vi "发送测试脚本.vi"(7 "Script Name":string="TSB_Script", 8 "错误输入":errorcluster, 10 "Script":string, 11 "VISA资源名称":refnum<visa-resource-name>) -> (0 "错误输出":errorcluster, 3 "VISA资源名称输出":refnum<visa-resource-name>)   [LabVIEW 2021]
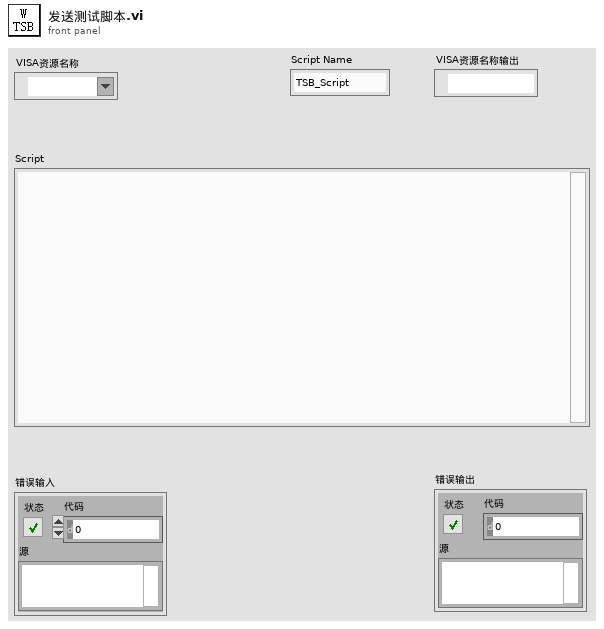
[diagram p1: front panel]
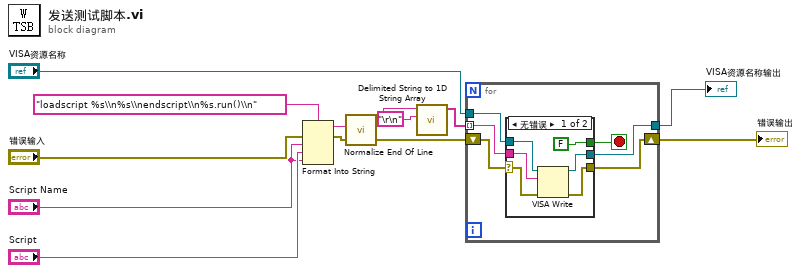
[diagram p0: block diagram]
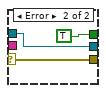
[diagram p2: hidden frame]
diagram:
  n1 = Format Into String(format string="loadscript %s\\n%s\\nendscript\\n%s.run()\\n", error in="错误输入", "Script Name", "Script", "Script Name") -> (resulting string=w4:string, error out=w1:errorcluster)  [unwired: 1 in]
  n2 = call <vilib>:"Normalize End Of Line.vi"("string in"=w4) -> ("string out"=w5:string)  [unwired: 7 in]
  n3 = call <vilib>:"Delimited String to 1D String Array.vi"("delimiter"="\r\n", "delimited string"=w5) -> ("string array"=w3:string[])  [unwired: 9 in]
  n4 = for {
    tunnel: "VISA资源名称" -> [w18]
    tunnel: [w16] -> w9
    shift-right: [w17] -> w8
    shift-left: w1 -> [w15]
    tunnel: w3 -> [w14] mode=indexing
    stop <- w13 stop-if-true
    n5 = case shown="无错误" w15 {
      selector: w15 -> [w21 w26]
      tunnel: [FALSE TRUE] -> w13
      tunnel: w18 -> [w24 w25]
      tunnel: [w23 w26] -> w17
      tunnel: [w22 w25] -> w16
      tunnel: w14 -> [w20 _]
      frame No Error {
        n6 = VISA Write(VISA resource name=w24, write buffer=w20, error in (no error)=w21) -> (VISA resource name out=w22:refnum<visa-resource-name>, error out=w23:errorcluster)  [unwired: 1 out]
      }
      frame Error {
      }
    }
  }
  "VISA资源名称输出" <- w9
  "错误输出" <- w8
